vi "Finalize To JSON 1.0.vi"(8 "error in (no error)":errorcluster, 11 "channel configuration 1.0":T1(array[cluster])) -> (0 "error out":errorcluster, 3 "json":string)   [LabVIEW 2017, in "DSF Core.lvlib" / "Core Channels Configuration.lvclass"]
uses:
  Core Channels Configuration.lvclass
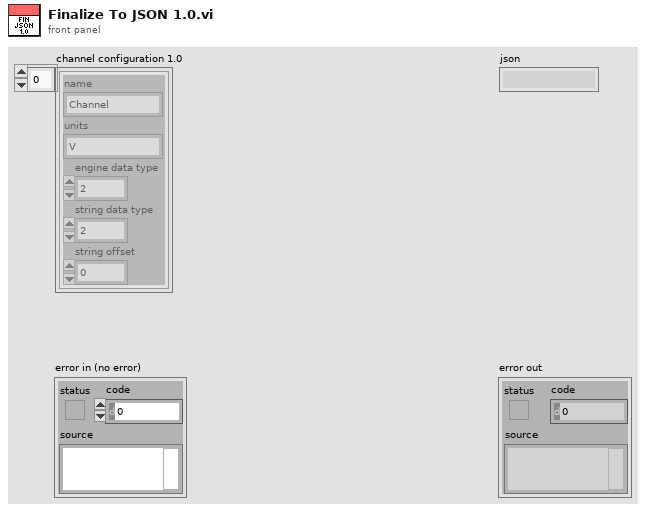
[diagram p1: front panel]
types:
  T1 = cluster{"name":string, "units":string, "engine data type":u8, "string data type":u8, "string offset":u64}[]
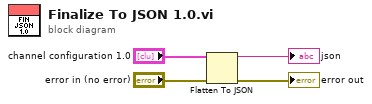
[diagram p0: block diagram]
diagram:
  n1 = Flatten To JSON(anything="channel configuration 1.0", error in (no error)="error in (no error)") -> (JSON string=→"json":string, 11:→"error out":errorcluster)  [unwired: 1 in]
